vi "TDS RF Power Input Offset.vi"(8 "error in (no error)":errorcluster, 9 "Offset":dbl, 10 "Signal InstConfig":string, 11 "Address":string) -> (0 "error out":errorcluster)   [LabVIEW 2025, in "Interface Functions.lvlib"]
uses:
  Interface Functions.lvlib
  <instrlib>/Agilent U2000 Series/Agilent U2000 Series.lvlib
panel:
  # "RF Power Input Offset"
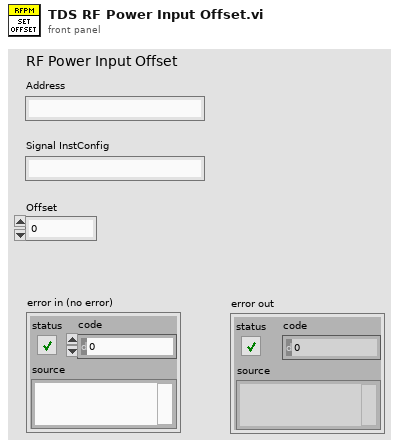
[diagram p1: front panel]
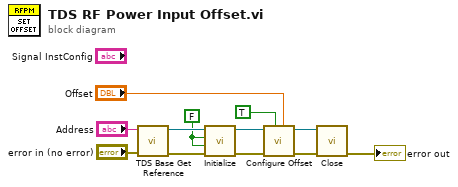
[diagram p0: block diagram]
diagram:
  w8 = FALSE ("ID Query (True)")
  n1 = call "TDS Base Get Reference.vi"("error in (no error)"="error in (no error)", "Address"="Address") -> ("error out"=w10:errorcluster, "Reference"=w9:refnum<visa-resource-name>)  [unwired: 8 in]
  n2 = call <instrlib>:"Initialize.vi"("error in (no error)"=w10, "Reset (True)"=w8, "ID Query (True)"=w8, "VISA resource name"=w9) -> ("error out"=w6:errorcluster, "VISA resource name out"=w5:refnum<visa-resource-name>)  [unwired: 6 in]
  n3 = call <instrlib>:"Configure Offset.vi"("Offset Value (0 dB)"="Offset", "Enable Offset (F: Disable)"=TRUE, "error in (no error)"=w6, "VISA resource name"=w5) -> ("error out"=w1:errorcluster, "VISA resource name out"=w2:refnum<visa-resource-name>)  [unwired: 6 in]
  n4 = call <instrlib>:"Close.vi"("error in (no error)"=w1, "VISA resource name"=w2) -> ("error out"=→"error out":errorcluster)  [unwired: 9 in]
